vi "catWalkArduinoNew.vi"() -> ()   [LabVIEW 2012]
uses:
  <vilib>/userdefined/High Color/IMAQdx.ctl
  <vilib>/Platform/TimedLoop/XDataNode/timing_clust.ctl
  <vilib>/Platform/TimedLoop/XDataNode/nitl_modes.ctl
  <vilib>/Platform/TimedLoop/XDataNode/wakeup.ctl
  XY Stage/XYStage.llb/GlobalXYStage.vi
  image acquisition/GlobalBaslerCamera.vi
  GlobalStatus.vi
  Cpp Libraries/CatWalkLabviewDLL/labview code/OpenCvGlobals.vi
  GlobalValves.vi
  GlobalLB.vi
  <vilib>/Platform/TimedLoop/XDataNode/XDataNode.xnode
  <vilib>/Platform/TimedLoop/XDataNode/XDNodeRunTimeDep.lvlib
panel:
  out "last time collected fly":u32=479694288
  out "manualStopIndicator":bool=TRUE caption="stop"
  in  "simulated LB status 5":bool[](array[boolean])=[FALSE, FALSE, FALSE, FALSE, FALSE, FALSE]
  in  "simulated LB status 4":bool[](array[boolean])=[FALSE, FALSE, FALSE, FALSE, FALSE, FALSE]
  in  "simulated LB status 3":bool[](array[boolean])=[FALSE, FALSE, FALSE, FALSE, FALSE, FALSE]
  in  "simulated LB status 2":bool[](array[boolean])=[FALSE, FALSE, FALSE, FALSE, FALSE, FALSE]
  in  "autoStop":bool
  in  "stop 2":bool
  in  "Image processing preferences":T1={"scale"=0.5, "elSizeImOpen"=21, "thresholdBinarizationBody"=0.5, "thresholdBinarizationWings"=0.12, "minWingArea"=20000, "quantile"=0.05, "elSizeImOpenIdent1"=15, "elSizeImOpenIdent2"=21, "thresholdBinarizationIdent"=0.65, "elSizeImHMin"=6, "raiseParImHMin"=0.33, "focus limit"=120, "maxAllowedRotation"=30.0, "elSizeImClose"=3, "numIterImClose"=3, "symmetryMinOverlapBody"=95.0, "symmetryMinOverlapWings"=80.0, "thresholdReflectionCheck"=0.99, "elSizeReflection"=7, "maxReflectionArea"=2000, "upSideDownCheck"=260.0}
  out "pre-processing result":T2(plugin-control)
  out "task out":T3(ring)
  out "task":bool=TRUE
  out "status":cluster{"Program status":u32, "message":string}={"Program status"=6618880, "message"="Ready"}
  out "measured flies":i32(slide) caption="Measured flies" scale=0.0..182.0
  out "stop indicator":bool=TRUE
  out "touching rigth border":bool
  in  "image selector":u16(ring) items=["raw image", "single channel", "focus check", "downsampled", "subtraction result", "thresholded", "filtered", "cleaned", "cropped"]
  out "acquiring video":bool
  out "acquired FPS":dbl
  out "processed FPS":dbl
  out "image":T2(plugin-control)
  out "saving background":bool
  in  "Robot Position":T4(radio)
  in  "system info":T5(tab)
  in  "minimum valid\nimages per fly":i32=3 min=1 max=10 step=1
  in  "max time\nin chamber (s)":u32=20
  out "light barriers":bool[](array[boolean])=[FALSE, TRUE]
  in  "loop period (ms)":i64=10
  out "resulting frequency (Hz)":dbl=100.0
  out "valves status":bool[](array[boolean])
  in  "resave BG time":u32=120
  in  "milliseconds to wait\nafter detection":u32
  in  "max number of\nimages per fly":i32=100
  in  "activate flies time interval (s)":u32=30
  out "done sorting":bool
  in  "sort one by one":bool
  in  "max time \nin chamber after\ndetection (s)":u32=25
  in  "inactivity alarm time interval (s)":u32=180
  in  "valve open time blow back":u32=1500
  in  "valve open time eject":u32=2000
  in  "valve open time keep":u32=5000
  in  "open valve":bool
  in  "valve close":bool[](array[boolean])=[FALSE, FALSE, FALSE, FALSE, FALSE, FALSE, FALSE, FALSE]
  in  "valve to hangar":bool[](array[boolean])=[TRUE, FALSE, TRUE, FALSE, FALSE, FALSE, FALSE, FALSE]
  in  "valve back":bool[](array[boolean])=[TRUE, FALSE, FALSE, FALSE, FALSE, FALSE, FALSE, FALSE]
  in  "valve eject":bool[](array[boolean])=[FALSE, TRUE, TRUE, FALSE, FALSE, FALSE, FALSE, FALSE]
  in  "valves puffed":bool[](array[boolean])=[FALSE, FALSE, TRUE, FALSE, FALSE, FALSE, FALSE, FALSE]
  in  "numPuffs keep":i32=3 min=1 max=10
  in  "numPuffs eject":i32=5
  in  "numPuffs blowback":i32=2 min=1 max=10
  in  "waitms before puff":u32=300
  in  "valve open time activate":u32=1000
  in  "number of\npuffs for scaring":i32=2
  in  "valve open time pre":u32=400
  in  "numPuffs eject pre":i32=3
  in  "valve open time blow back 2":u32=1000
  in  "valve open time activate pre":u32=1000
  in  "USB COM port":refnum<visa-resource-name>="COM3"
  in  "robot limits":T6={"xmin"=-16850, "xmax"=-1660, "ymin"=-15485, "ymax"=-550}
  in  "Motor high speed":i32=5000
  in  "Motor low speed":i32=100
  in  "Motor acc":i32=500
  in  "gate 0 closed blowing":u16=1380
  in  "fly trap open":u16=1490
  in  "fly trap close":u16=1490
  in  "fly ejector open":u16=1350
  in  "fly ejector close":u16=900
  in  "fly sieve hangar":u16=1390
  in  "gate 0 closed":u16=1390
  in  "gate 0 open":u16=1470
  in  "fly sieve back":u16=1680
  in  "fly sieve odour":u16=1140
  in  "bottle positions":u16[](array[numeric])=[1115, 1210, 1290]
  in  "shakeSpan":i8 max=63 step=1
  in  "gate 0 open blowing":u16=1470
  in  "free gate after keeping":bool=TRUE
  in  "disable servo delay (ms)":u32=200
  in  "fly ejector semi close":u16=1150
  in  "numShakes":i32=3
  in  "shake speed":u32=50
  in  "insensitivity time (ms)":u32=2000
  in  "camera controls":T8={"Camera Name"="cam0", "exposure time (us)"=600, "GainRaw"=200, "Red balance"=75, "Green balance"=80, "Blue balance"=64}
  in  "image format controls":T9={"Pixel Format"="YUV 422 Packed", "width"=2448, "height"=900, "sub image height"=600, "sub image width"=1500}
  in  "im proc controls":T10={"Color Plane"=2, "downsampling"=64, "Filter"=enum."AutoM", "Number of Erosions"=1, "Focus threshold"=20.0, "Focus std threshold"=0.0, "background\nsubtraction"=TRUE, "Threshold"=40} {"Threshold" scale=0.0..255.0; "downsampling" min=1 max=128; "Color Plane" items=["Red", "Green", "Blue", "Hue", "Saturation", "Luminance", "Value", "Intensity"]}
  in  "adjust image":bool
  out "filled buffer":i32(slide) max=20 scale=0.0..500.0
  in  "buffer size":i32=500
  in  "simulate LB":bool
  in  "simulated LB status":bool[](array[boolean])=[FALSE, FALSE, FALSE, FALSE, FALSE, FALSE]
  out "events check loop":i32=163273
  in  "debugOpenCV":bool
  in  "keep all flies":bool
  out "numCycles":i32=198986
  in  "experiment name":string="L1S4fb"
  in  "data path":path=path "Y:/WingXDataRemote"
  in  "temp path":path=path "C:/wingXTemp"
  in  "sounds":T11={"welcome sound"=path "C:/Users/wingX/Documents/WingXSVN/labview/daq test/sounds/welcome.wav", "play welcome"=FALSE, "got fly sound"=path "C:/Users/wingX/Documents/WingXSVN/labview/daq test/sounds/gotFly.wav", "play got fly"=FALSE, "discard sound"=path "C:/Users/wingX/Documents/WingXSVN/labview/daq test/sounds/blowingback.wav", "play discard"=FALSE, "finish sound"=path "C:/Users/wingX/Documents/WingXSVN/labview/daq test/sounds/done.wav", "play finish"=TRUE, "inactivity alarm sound"=path "C:/Users/wingX/Documents/WingXSVN/labview/daq test/sounds/inactivity.wav", "play inactivity\nalarm"=TRUE}
  in  "stop":bool
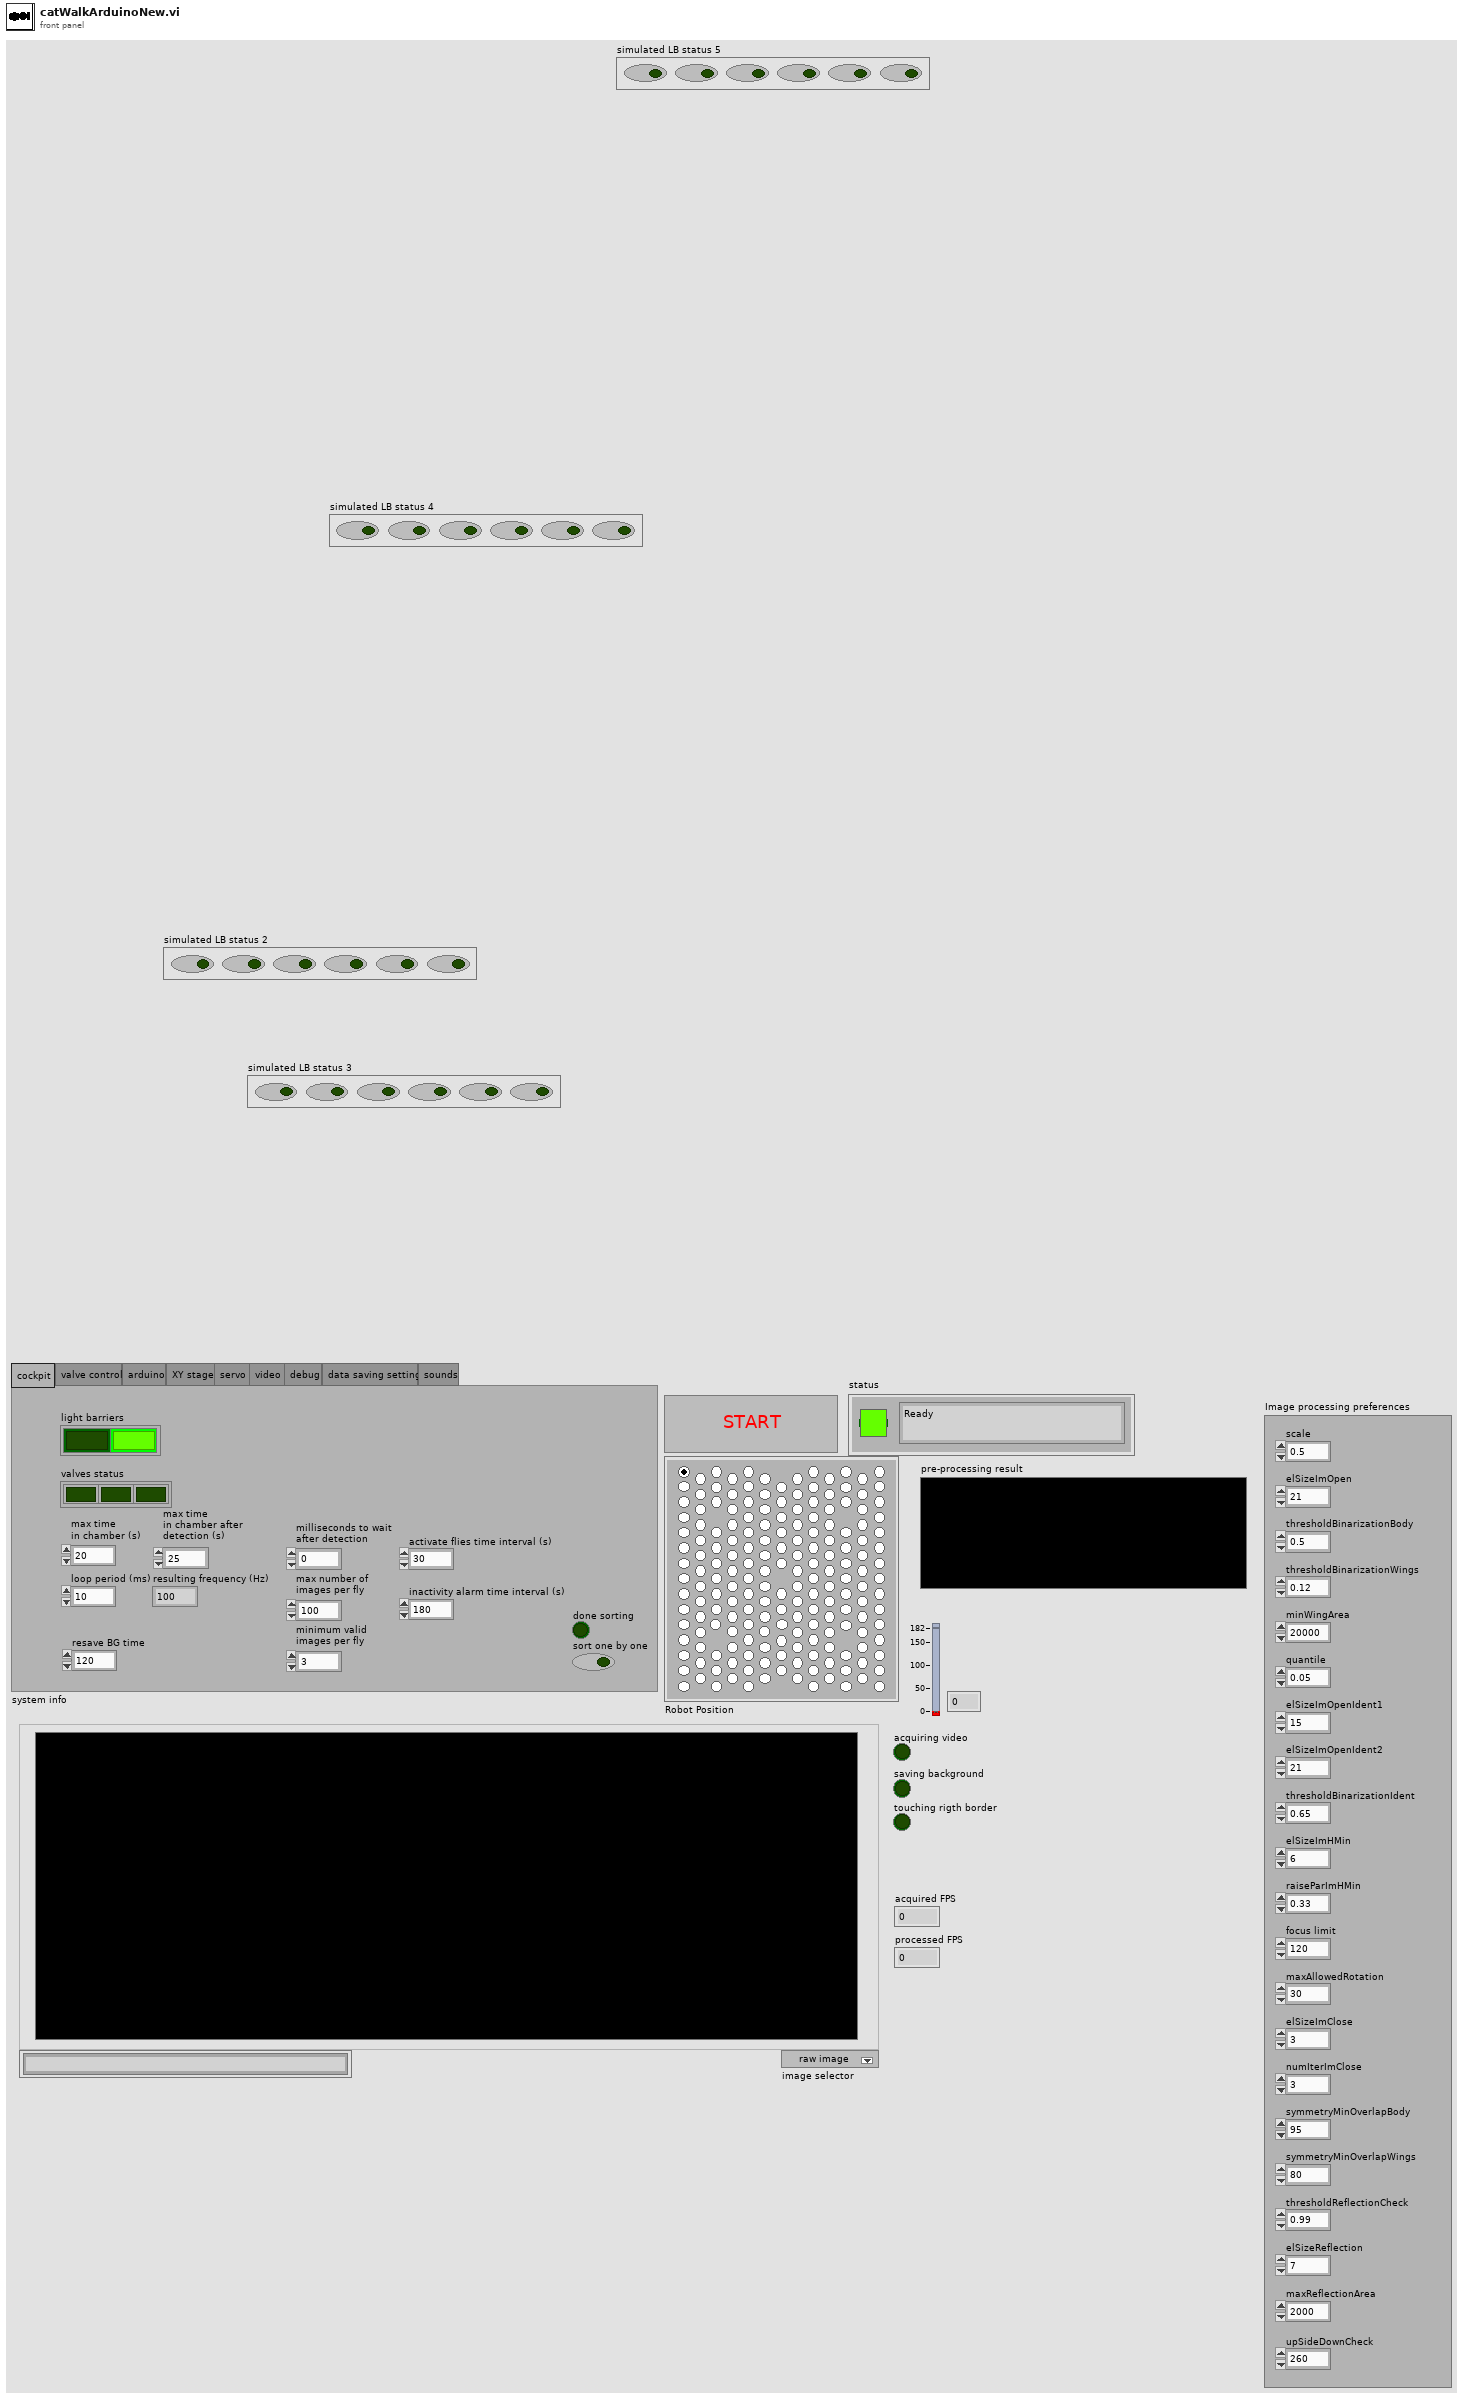
[diagram p1: front panel]
types:
  T1 = cluster{"scale":sgl, "elSizeImOpen":i32, "thresholdBinarizationBody":sgl, "thresholdBinarizationWings":sgl, "minWingArea":i32, "quantile":sgl, "elSizeImOpenIdent1":i32, "elSizeImOpenIdent2":i32, "thresholdBinarizationIdent":sgl, "elSizeImHMin":i32, "raiseParImHMin":sgl, "focus limit":i32, "maxAllowedRotation":sgl, "elSizeImClose":i32, "numIterImClose":i32, "symmetryMinOverlapBody":sgl, "symmetryMinOverlapWings":sgl, "thresholdReflectionCheck":sgl, "elSizeReflection":i32, "maxReflectionArea":i32, "upSideDownCheck":sgl}
  T2 = typedef "IMAQ Image.ctl" = refnum<image>
  T3 = enum16{"waiting for fly", "closing gate", "fly in chamber", "taking decision", "keeping the fly", "blowing back", "activate flies"}
  T4 = enum32{"Radio Selection 1", "Radio Selection 2", "Radio Selection 3", "Radio Selection 5", "Radio Selection 6", "Radio Selection 8", "Radio Selection 13", "Radio Selection 14", "Radio Selection 15", "Radio Selection 16", "Radio Selection 17", "Radio Selection 18", "Radio Selection 7", "Radio Selection 9", "Radio Selection 10", "Radio Selection 11", "Radio Selection 12", "Radio Selection 19", "Radio Selection 20", "Radio Selection 21", "Radio Selection 22", "Radio Selection 23", "Radio Selection 24", "Radio Selection 25", "Radio Selection 26", "Radio Selection 27", "Radio Selection 28", "Radio Selection 29", "Radio Selection 30", "Radio Selection 31", "Radio Selection 32", "Radio Selection 33", "Radio Selection 34", "Radio Selection 35", "Radio Selection 36", "Radio Selection 37", "Radio Selection 38", "Radio Selection 39", "Radio Selection 40", "Radio Selection 42", "Radio Selection 43", "Radio Selection 44", "Radio Selection 46", "Radio Selection 41", "Radio Selection 45", "Radio Selection 47", "Radio Selection 48", "Radio Selection 49", "Radio Selection 50", "Radio Selection 51", "Radio Selection 52", "Radio Selection 53", "Radio Selection 54", "Radio Selection 55", "Radio Selection 56", "Radio Selection 57", "Radio Selection 58", "Radio Selection 59", "Radio Selection 60", "Radio Selection 61", "Radio Selection 62", "Radio Selection 63", "Radio Selection 64", "Radio Selection 65", "Radio Selection 66", "Radio Selection 67", "Radio Selection 68", "Radio Selection 69", "Radio Selection 70", "Radio Selection 71", "Radio Selection 72", "Radio Selection 73", "Radio Selection 74", "Radio Selection 75", "Radio Selection 76", "Radio Selection 77", "Radio Selection 78", "Radio Selection 79", "Radio Selection 80", "Radio Selection 81", "Radio Selection 82", "Radio Selection 83", "Radio Selection 84", "Radio Selection 85", "Radio Selection 86", "Radio Selection 87", "Radio Selection 88", "Radio Selection 89", "Radio Selection 4", "Radio Selection 90", "Radio Selection 91", "Radio Selection 92", "Radio Selection 93", "Radio Selection 94", "Radio Selection 95", "Radio Selection 96", "Radio Selection 97", "Radio Selection 98", "Radio Selection 99", "Radio Selection 100", "Radio Selection 101", "Radio Selection 102", "Radio Selection 103", "Radio Selection 104", "Radio Selection 105", "Radio Selection 106", "Radio Selection 107", "Radio Selection 108", "Radio Selection 109", "Radio Selection 110", "Radio Selection 111", "Radio Selection 112", "Radio Selection 113", "Radio Selection 114", "Radio Selection 115", "Radio Selection 116", "Radio Selection 117", "Radio Selection 118", "Radio Selection 119", "Radio Selection 120", "Radio Selection 121", "Radio Selection 122", "Radio Selection 123", "Radio Selection 124", "Radio Selection 125", "Radio Selection 126", "Radio Selection 127", "Radio Selection 128", "Radio Selection 129", "Radio Selection 130", "Radio Selection 131", "Radio Selection 132", "Radio Selection 133", "Radio Selection 134", "Radio Selection 135", "Radio Selection 136", "Radio Selection 137", "Radio Selection 138", "Radio Selection 139", "Radio Selection 140", "Radio Selection 141", "Radio Selection 142", "Radio Selection 143", "Radio Selection 144", "Radio Selection 145", "Radio Selection 146", "Radio Selection 147", "Radio Selection 148", "Radio Selection 149", "Radio Selection 150", "Radio Selection 151", "Radio Selection 152", "Radio Selection 153", "Radio Selection 154", "Radio Selection 155", "Radio Selection 156", "Radio Selection 157", "Radio Selection 158", "Radio Selection 159", "Radio Selection 160", "Radio Selection 161", "Radio Selection 162", "Radio Selection 163", "Radio Selection 164", "Radio Selection 165", "Radio Selection 166", "Radio Selection 167", "Radio Selection 168", "Radio Selection 169", "Radio Selection 170", "Radio Selection 171", "Radio Selection 172", "Radio Selection 173", "Radio Selection 174", "Radio Selection 175", "Radio Selection 176", "Radio Selection 177", "Radio Selection 178", "Radio Selection 179", "Radio Selection 180", "Radio Selection 181", "Radio Selection 182"}
  T5 = enum32{"cockpit", "valve control", "arduino", "XY stage", "servo", "video", "debug", "data saving settings", "sounds"}
  T6 = cluster{"xmin":i32, "xmax":i32, "ymin":i32, "ymax":i32}
  T7 = typedef "IMAQdx.ctl" = refnum<k21>
  T8 = cluster{"Camera Name":T7, "exposure time (us)":u32, "GainRaw":i64, "Red balance":i64, "Green balance":i64, "Blue balance":i64}
  T9 = cluster{"Pixel Format":string, "width":u32, "height":u32, "sub image height":u32, "sub image width":u32}
  T10 = cluster{"Color Plane":i32, "downsampling":i32, "Filter":enum32{"AutoM", "Close", "Dilate", "Erode", "Gradient", "Gradient out", "Gradient in", "Hit miss", "Open", "PClose", "POpen", "Thick", "Thin"}, "Number of Erosions":i32, "Focus threshold":sgl, "Focus std threshold":sgl, "background\nsubtraction":bool, "Threshold":u8}
  T11 = cluster{"welcome sound":path, "play welcome":bool, "got fly sound":path, "play got fly":bool, "discard sound":path, "play discard":bool, "finish sound":path, "play finish":bool, "inactivity alarm sound":path, "play inactivity\nalarm":bool}
  T12 = typedef "XDNodeRunTimeDep.lvlib/timing_clust.ctl" = cluster{"Expected End [f-1]":u64, "Actual End [f-1]":u64, "Finished Late? [f-1]":bool, "Expected End [i-1]":u64, "Actual End [i-1]":u64, "Finished Late? [i-1]":bool, "Expected Start [i]":u64, "Actual Start [i]":u64, "Expected Start [f]":u64, "Actual Start [f]":u64, "Source Name":string, "Structure Name":string, "Period":i64, "Deadline":i64, "Offset":i64, "Start":i64, "Priority":i32, "Timeout":i32, "Mode":T13, "Wakeup Reason":T14, "Error":errorcluster, "Source Type":string, "Secondary Source Type":string, "Global End Time":u64, "Global Start Time":u64, "Frame Duration":u64, "Iteration Duration":u64, "Assigned CPU":i32, "I/O Scan Engine Mode":u32}
  T13 = typedef "XDNodeRunTimeDep.lvlib/nitl_modes.ctl" = enum32{"No Change", "Process missed periods, maintain original phase", "Discard missed periods, maintain original phase", "Process missed periods, ignore original phase", "Discard missed periods, ignore original phase"}
  T14 = typedef "XDNodeRunTimeDep.lvlib/wakeup.ctl" = enum32{"Normal", "Aborted", "Asynchronous wakeup", "Timing source error", "Timed loop error", "Timeout"}
  T15 = enum16{"Left Button", "Center Button", "Right Button", "Window Close"}
  T16 = typedef "Semaphore RefNum" = refnum<k1>
  T17 = enum8{"Enabled", "Disabled", "Disabled and Grayed Out"}
  T18 = cluster{"raw":T2, "single channel":T2, "focus check":T2, "downsampled":T2, "subtraction":T2, "thresholded":T2, "filtered":T2, "cleaned":T2, "cropped":T2}
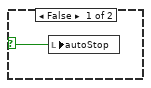
[diagram p2: hidden frame]
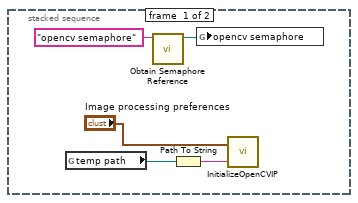
[diagram p4: hidden frame]
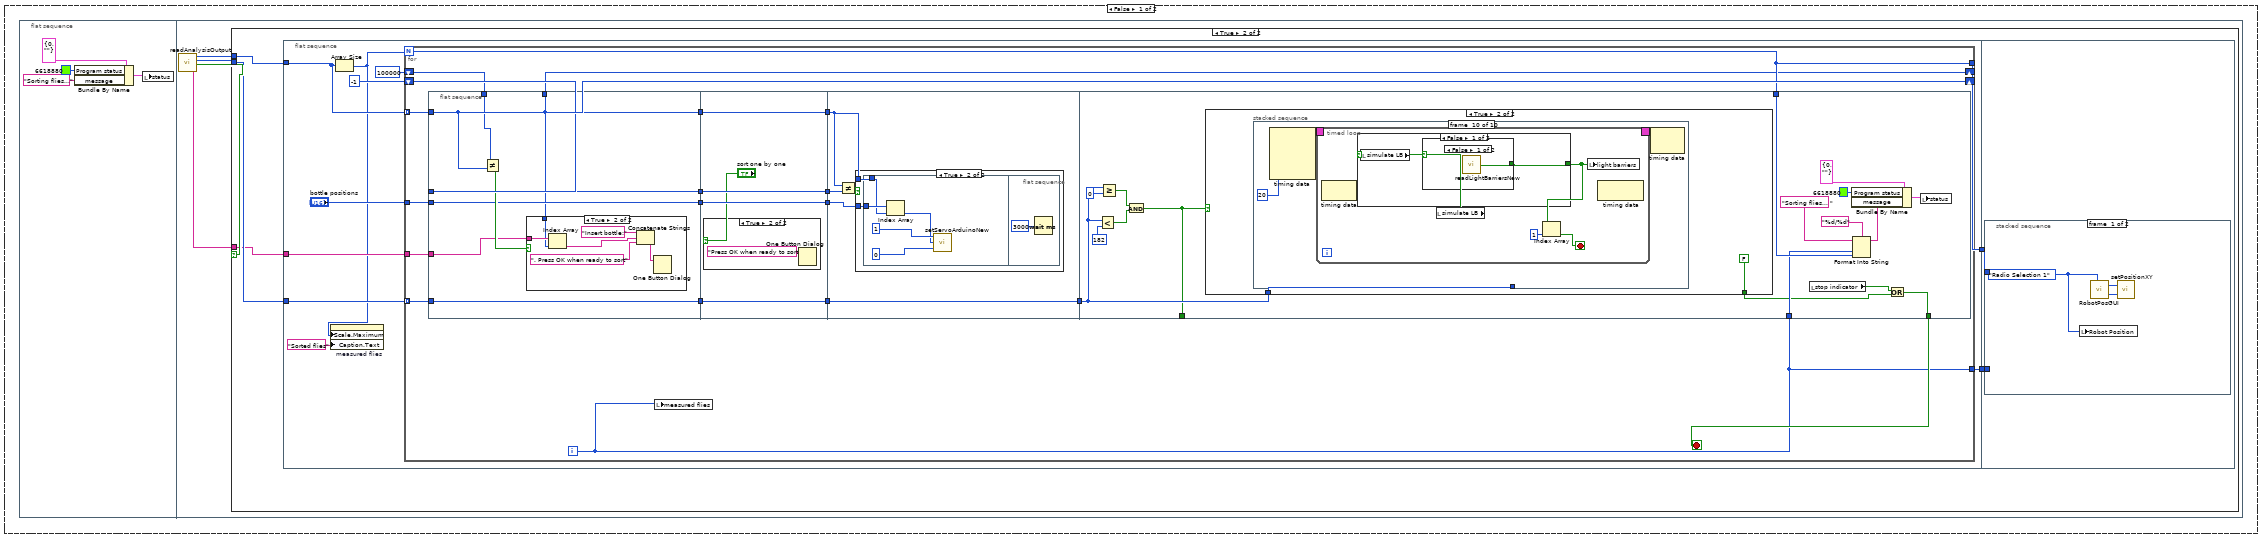
[diagram p6: hidden frame]
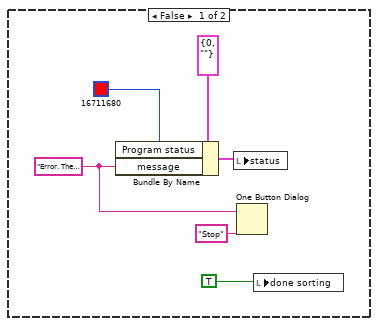
[diagram p7: hidden frame]
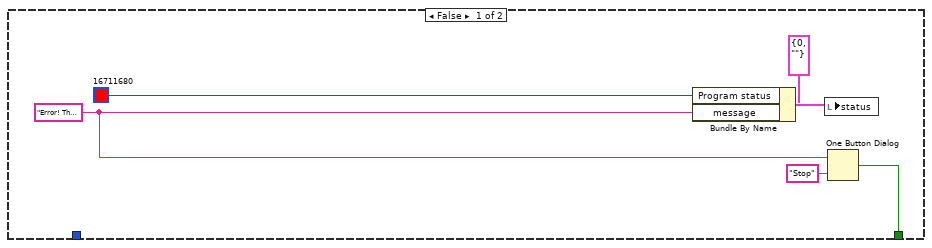
[diagram p11: hidden frame]
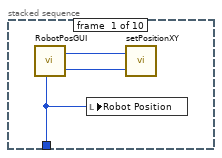
[diagram p12: hidden frame]
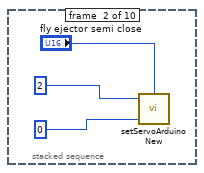
[diagram p13: hidden frame]
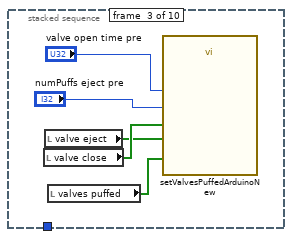
[diagram p14: hidden frame]
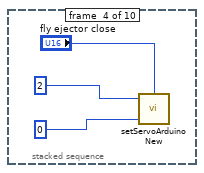
[diagram p15: hidden frame]
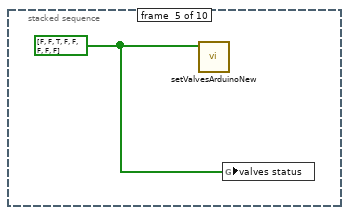
[diagram p16: hidden frame]
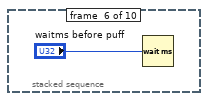
[diagram p17: hidden frame]
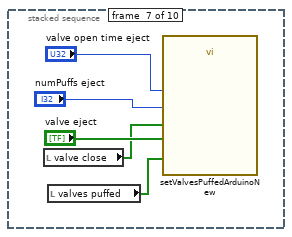
[diagram p18: hidden frame]
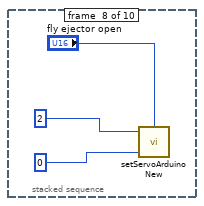
[diagram p19: hidden frame]
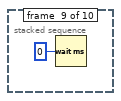
[diagram p20: hidden frame]
diagram:
  n1 = while {
    stop <- "stop 2" stop-if-true
    n2 = flat-sequence {
      tunnel: ["loop period (ms)"] -> w3
      tunnel: w3 -> [w80]
      tunnel: [w80] -> w2
      tunnel: w2 -> [w85]
      frame #0 {
        n3 = node-c288(i64 10 ("Period")) -> (w10:T12)  [unwired: 3 in]
        n4 = timed-loop {
          timing: w10 -> [_]
          timing-out: [_] -> w9
          stop <- w13 stop-if-true
          n5 = node-c288() -> ()  [unwired: 1 in, 1 out]
          n6 = local read "Robot Position"() -> (w12:T4)
          n7 = global write "GlobalXYStage.vi" "Robot Position"(w12) -> ()
          n8 = local write "measured flies"(w12) -> ()
          n9 = local read "stop"() -> (w13:bool)
          n10 = node-c288() -> ()  [unwired: 1 in, 1 out]
        }
        n11 = property on="stop" class="Bool (strict)"("BoolText.Text"="START" ("Boolean Text.Text")) -> ()  [unwired: 2 in, 2 out]
        n12 = Bundle By Name(cluster=cluster{"Program status":u32, "message":string} {"Program status"=0, "message"=""} ("status 2"), "Program status"=u32 6618880, "message"="Ready") -> (w5:cluster{"Program status":u32, "message":string})
        n13 = local write "status"(w5) -> ()
        n14 = node-c288(w9) -> ()  [unwired: 1 out]
      }
      frame #1 {
        w20 = FALSE ("stop indicator")
        # "init arduino and close gate"
        n15 = flat-sequence {
          frame #0 {
            n16 = call "initArduinoNew.vi"("VISA resource"="USB COM port") -> ()
          }
          frame #1 {
            n17 = local read "fly ejector open"() -> (w30:u16)
            n18 = local read "gate 0 closed"() -> (w35:u16)
            n19 = call "setServoArduinoNew.vi"("speed"=u8 0, "Pulse Width in uS"=w35, "servo id"=u8 0 ("channel")) -> ()
            n20 = call "setServoArduinoNew.vi"("speed"=u8 0, "Pulse Width in uS"=w30, "servo id"=u8 2 ("channel")) -> ()
          }
          frame #2 {
            n21 = Wait (ms)(milliseconds to wait=u32 500) -> ()  [unwired: 1 out]
          }
          frame #3 {
            n22 = call "disableServosArduinoNew.vi"() -> ()  [unwired: 1 in]
          }
        }
        n23 = property on="stop" class="Bool (strict)"("Value"=FALSE ("stop")) -> ()  [unwired: 2 in, 2 out]
        n24 = property on="stop" class="Bool (strict)"("BoolText.Text"="STOP" ("Boolean Text.Text")) -> ()  [unwired: 2 in, 2 out]
        n25 = local write "stop indicator"(w20) -> ()
        n26 = Bundle By Name(cluster=cluster{"Program status":u32, "message":string} {"Program status"=0, "message"=""} ("status 2"), "Program status"=u32 16776960, "message"="Initializing...") -> (→"status":cluster{"Program status":u32, "message":string})
        n27 = property on="measured flies" class="Slide (strict)"("Scale.Maximum"=182 ("Scale.Range:Maximum"), "Caption.Text"="") -> ()  [unwired: 2 in, 2 out]
        "done sorting" <- w20
      }
      frame #2 {
        n28 = local read "adjust image"() -> (w54:bool)
        n29 = global write "GlobalBaslerCamera.vi" "temp path"("temp path") -> ()
        n30 = global write "GlobalBaslerCamera.vi" "data path"("data path") -> ()
        n31 = Divide(x=i64 1000, y="loop period (ms)") -> (x/y=→"resulting frequency (Hz)":dbl)
        n32 = call <vilib>:"Three Button Dialog.vi"("Right Button Text (\"Cancel\")"="Sort Flies" ("F button name (\"Cancel\")"), "Center Button Text (\"No\")"="Measure flies starting from current position" ("T button name (\"OK\")"), "Left Button Text (\"Yes\")"="Measure flies" ("T button name (\"OK\")"), "message"="WELCOME TO THE FLY CATWALK\n\nWhat do you want to do?") -> ("Which Button?"=w38:T15)  [unwired: 7 in]
        n33 = Equal?(x=T15."Center Button", y=w38) -> (x = y?=w42:bool)
        n34 = global write "GlobalBaslerCamera.vi" "adjust image"(w54) -> ()
        n35 = call "initXYStage.vi"("Motor high speed"="Motor high speed", "restart from\ncurrent position"=w42, "Motor acc"="Motor acc", "Motor low speed"="Motor low speed", "robot limits"="robot limits") -> ("Robot Position"=w40:T4)
        "measured flies" <- w40
        n36 = global write "GlobalStatus.vi" "hangar full"(FALSE ("hangar full")) -> ()
        n37 = Less?(x=w38, y=T15."Right Button") -> (x < y?=w44:bool)
        "task" <- w44
        n38 = case shown="True" w44 {
          frame False {
          }
          frame True {
            n39 = stacked-sequence {
              frame #0 {
                n40 = global read "GlobalBaslerCamera.vi" "temp path"() -> (w67:path)
                n41 = call <vilib>:"Obtain Semaphore Reference.vi"("name (unnamed)"="opencv semaphore") -> ("semaphore"=w64:T16)  [unwired: 4 in, 2 out]
                n42 = Path To String(path=w67) -> (string=w66:string)
                n43 = global write "OpenCvGlobals.vi" "opencv semaphore"(w64) -> ()
                n44 = call "InitializeOpenCVIP.vi"("dataDirectory"=w66, "Image processing preferences"="Image processing preferences") -> ()  [unwired: 1 out]
              }
              frame #1 {
                n45 = local read "im proc controls"() -> (w69:T10)
                n46 = call "initBaslerCamera.vi"("buffer size"="buffer size", "camera controls"="camera controls", "im proc controls"=w69, "image format controls"="image format controls") -> ()  [unwired: 4 in]
                n47 = property on="filled buffer" class="Slide (strict)"("Scale.Maximum"="buffer size") -> ()  [unwired: 2 in, 2 out]
              }
            }
          }
        }
        n48 = Equal?(x=T15."Window Close", y=w38) -> (x = y?=w39:bool)
        n49 = global write "GlobalBaslerCamera.vi" "experiment name"("experiment name") -> ()
        n50 = case shown="True" w39 {
          selector: w39 -> [w61 w62]
          frame False {
            n51 = local write "autoStop"(w61) -> ()
          }
          frame True {
            n52 = local write "autoStop"(w62) -> ()
          }
        }
        n53 = local write "Robot Position"(w40) -> ()
      }
      frame #3 {
        w79 = T17."Disabled and Grayed Out" ("Disabled")
        n54 = global write "OpenCvGlobals.vi" "isDebug"("debugOpenCV") -> ()
        n55 = local read "fly sieve odour"() -> (w76:u16)
        n56 = local read "gate 0 closed"() -> (w72:u16)
        n57 = property on="loop period (ms)" class="DigNum (strict)"("DisabledEnum"=w79) -> ()  [unwired: 2 in, 2 out]
        n58 = property on="image format controls" class="Clust (strict)"("DisabledEnum"=w79) -> ()  [unwired: 2 in, 2 out]
        n59 = property on="camera controls" class="Clust (strict)"("DisabledEnum"=w79) -> ()  [unwired: 2 in, 2 out]
        n60 = property on="temp path" class="Path"("DisabledEnum"=w79) -> ()  [unwired: 2 in, 2 out]
        n61 = property on="data path" class="Path"("DisabledEnum"=w79) -> ()  [unwired: 2 in, 2 out]
        n62 = call "setServoArduinoNew.vi"("speed"=u8 0, "Pulse Width in uS"=w76, "servo id"=u8 1 ("channel")) -> ()
        n63 = call "setServoArduinoNew.vi"("speed"=u8 0, "Pulse Width in uS"=w72, "servo id"=u8 0 ("channel")) -> ()
      }
      frame #4 {
        n64 = node-c288(i64 100 ("Period")) -> (w84:T12)  [unwired: 3 in]
        n65 = local read "task"() -> (w81:bool)
        n66 = timed-loop {
          timing: w84 -> [_]
          timing-out: [_] -> w83
          stop <- w92 stop-if-true
          n67 = node-c288() -> ()  [unwired: 1 in, 1 out]
          n68 = local read "done sorting"() -> (w89:bool)
          n69 = global read "GlobalStatus.vi" "hangar full"() -> (w90:bool)
          n70 = Compound Arithmetic op=OR("autoStop", w90, w89, "stop") -> (w92:bool)
          "stop indicator" <- w92
          n71 = call "disableServosArduinoNew.vi"("delay (ms)"="disable servo delay (ms)") -> ()
          n72 = node-c288() -> ()  [unwired: 1 in, 1 out]
          "manualStopIndicator" <- "stop"
        }
        n73 = case shown="True" w81 {
          frame False {
          }
          frame True {
            n74 = property on="measured flies" class="Slide (strict)"("Caption.Text"="Measured flies" ("Label.Text")) -> ()  [unwired: 2 in, 2 out]
          }
        }
        n75 = node-c288(w83) -> ()  [unwired: 1 out]
        n76 = case shown="True" w81 {
          tunnel: w85 -> [_ w269]
          frame False {
            n77 = flat-sequence {
              frame #0 {
                n78 = Bundle By Name(cluster=cluster{"Program status":u32, "message":string} {"Program status"=0, "message"=""} ("status 2"), "Program status"=u32 6618880, "message"="Sorting flies...") -> (w100:cluster{"Program status":u32, "message":string})
                n79 = local write "status"(w100) -> ()
              }
              frame #1 {
                n80 = call "readAnalysisOutput.vi"() -> ("bottle number"=w106:i64[], "fly number"=w105:i64[], "folder exists"=w104:bool, "bottle label"=w103:string[])  [unwired: 1 in]
                n81 = case shown="True" w104 {
                  tunnel: w106 -> [_ w117]
                  tunnel: w105 -> [_ w116]
                  tunnel: w103 -> [_ w113]
                  frame False {
                    w109 = "Error. The selected directory does not contain an Analysisoutpu.txt file. It may not be analized yet. The program will stop immediately" ("message")
                    n82 = Bundle By Name(cluster=cluster{"Program status":u32, "message":string} {"Program status"=0, "message"=""} ("status 2"), "Program status"=u32 16711680, "message"=w109) -> (w111:cluster{"Program status":u32, "message":string})
                    n83 = local write "status"(w111) -> ()
                    n84 = One Button Dialog(message=w109, button name ("OK")="Stop") -> ()  [unwired: 1 out]
                    n85 = local write "done sorting"(TRUE) -> ()
                  }
                  frame True {
                    n86 = flat-sequence {
                      tunnel: w117 -> [w127]
                      tunnel: w116 -> [w124]
                      tunnel: [w123] -> w115
                      tunnel: [w122] -> w114
                      tunnel: w113 -> [w121]
                      tunnel: w115 -> [w248]
                      tunnel: w114 -> [w247]
                      frame #0 {
                        n87 = Array Size(array=w127) -> (size(s)=w119:i32)
                        n88 = property on="measured flies" class="Slide (strict)"("Scale.Maximum"=w119, "Caption.Text"="Sorted flies" ("Label.Text")) -> ()  [unwired: 2 in, 2 out]
                        n89 = for {
                          N: w119 -> [w141]
                          tunnel: w127 -> [w146] mode=indexing
                          shift-right: [w146] -> _
                          shift-left: i64 -1 -> [w145]
                          tunnel: "bottle positions" -> [w144]
                          tunnel: w124 -> [w142] mode=indexing
                          tunnel: [w128] -> w123
                          tunnel: [w141] -> w122
                          shift-right: [w129] -> _
                          shift-left: i64 100000 -> [w131]
                          tunnel: w121 -> [w130]
                          i -> [w128]
                          stop <- w136 stop-if-true
                          n90 = flat-sequence {
                            tunnel: w142 -> [w148]
                            tunnel: w144 -> [w149]
                            tunnel: w145 -> [w153]
                            tunnel: w146 -> [w147]
                            tunnel: [w147] -> w135
                            tunnel: [w153] -> w134
                            tunnel: [w149] -> w133
                            tunnel: [w148] -> w132
                            tunnel: w131 -> [w152]
                            tunnel: w130 -> [w150]
                            tunnel: [w147] -> w129
                            tunnel: [w164] -> w140
                            tunnel: [w163] -> w139
                            tunnel: [w162] -> w138
                            tunnel: [w161] -> w137
                            tunnel: w135 -> [w164]
                            tunnel: w134 -> [w163]
                            tunnel: w133 -> [w162]
                            tunnel: w132 -> [w161]
                            tunnel: [w166] -> w143
                            tunnel: w140 -> [w167]
                            tunnel: w139 -> [w169]
                            tunnel: w138 -> [w168]
                            tunnel: w137 -> [w166]
                            tunnel: [w190] -> _
                            tunnel: w143 -> [w194]
                            tunnel: w128 -> [w182]
                            tunnel: w141 -> [w185]
                            tunnel: [w179] -> w136
                            frame #0 {
                              n91 = Not Equal?(x=w152, y=w147) -> (x != y?=w151:bool)
                              n92 = case shown="True" w151 {
                                tunnel: w150 -> [_ w157]
                                tunnel: w147 -> [_ w156]
                                frame False {
                                }
                                frame True {
                                n93 = Index Array(array=w157, index=w156) -> (element=w155:string)
                                n94 = Concatenate Strings("Insert bottle:" ("message"), w155, ". Press OK when ready to sort" ("message")) -> (w154:string)
                                n95 = One Button Dialog(message=w154) -> ()  [unwired: 1 in, 1 out]
                                }
                              }
                            }
                            frame #1 {
                              n96 = case shown="True" "sort one by one" {
                                frame False {
                                }
                                frame True {
                                n97 = One Button Dialog(message="Press OK when ready to sort") -> ()  [unwired: 1 in, 1 out]
                                }
                              }
                            }
                            frame #2 {
                              n98 = Not Equal?(x=w167, y=w169) -> (x != y?=w170:bool)
                              n99 = case shown="True" w170 {
                                tunnel: w168 -> [_ w172]
                                tunnel: w167 -> [_ w171]
                                frame False {
                                }
                                frame True {
                                n100 = flat-sequence {
                                tunnel: w172 -> [w175]
                                tunnel: w171 -> [w174]
                                frame #0 {
                                n101 = Index Array(array=w175, index=w174) -> (element=w173:u16)
                                n102 = call "setServoArduinoNew.vi"("speed"=u8 0, "Pulse Width in uS"=w173, "servo id"=u8 1 ("channel")) -> ()
                                }
                                frame #1 {
                                n103 = Wait (ms)(milliseconds to wait=u32 3000) -> ()  [unwired: 1 out]
                                }
                                }
                                }
                              }
                            }
                            frame #3 {
                              n104 = Less?(x=w194, y=i64 182) -> (x < y?=w192:bool)
                              n105 = Greater Or Equal?(x=w194, y=i64 0) -> (x >= y?=w191:bool)
                              n106 = And(x=w191, y=w192) -> (x .and. y?=w190:bool)
                              n107 = case shown="True" w190 {
                                tunnel: w194 -> [_ w203]
                                tunnel: [w196 FALSE ("true")] -> w181
                                frame False {
                                w198 = "Error! The analysis output file contains invalid data.  The program will terminate immediately." ("message")
                                n108 = Bundle By Name(cluster=cluster{"Program status":u32, "message":string} {"Program status"=0, "message"=""} ("status 2"), "Program status"=u32 16711680, "message"=w198) -> (w200:cluster{"Program status":u32, "message":string})
                                n109 = local write "status"(w200) -> ()
                                n110 = One Button Dialog(message=w198, button name ("OK")="Stop") -> (true=w196:bool)
                                }
                                frame True {
                                n111 = stacked-sequence {
                                tunnel: w203 -> [w204 _ _ _ _ _ _ _ _ _]
                                frame #0 {
                                n112 = call "RobotPosGUI.vi"("Robot Position"=w204) -> ("X position"=w206:i32, "Y position"=w205:i32)  [unwired: 4 in]
                                n113 = local write "Robot Position"(w204) -> ()
                                n114 = call "setPositionXY.vi"("Y Position"=w205, "X Position"=w206) -> ()  [unwired: 1 in]
                                }
                                frame #1 {
                                n115 = call "setServoArduinoNew.vi"("speed"=u8 0, "Pulse Width in uS"="fly ejector semi close", "servo id"=u8 2 ("channel")) -> ()
                                }
                                frame #2 {
                                n116 = local read "valve close"() -> (w213:bool[])
                                n117 = local read "valve eject"() -> (w210:bool[])
                                n118 = local read "valves puffed"() -> (w212:bool[])
                                n119 = call "setValvesPuffedArduinoNew.vi"("valve data puffed"=w212, "valve data close"=w213, "valve data open"=w210, "milliseconds to wait"="valve open time pre", "numPuffs"="numPuffs eject pre") -> ()  [unwired: 7 in]
                                }
                                frame #3 {
                                n120 = call "setServoArduinoNew.vi"("speed"=u8 0, "Pulse Width in uS"="fly ejector close", "servo id"=u8 2 ("channel")) -> ()
                                }
                                frame #4 {
                                w218 = bool[] [FALSE, FALSE, TRUE, FALSE, FALSE, FALSE, FALSE, FALSE] ("valve data open")
                                n121 = call "setValvesArduinoNew.vi"("valve data"=w218) -> ()  [unwired: 11 in]
                                n122 = global write "GlobalValves.vi" "valves status"(w218) -> ()
                                }
                                frame #5 {
                                n123 = Wait (ms)(milliseconds to wait="waitms before puff") -> ()  [unwired: 1 out]
                                }
                                frame #6 {
                                n124 = local read "valve close"() -> (w222:bool[])
                                n125 = local read "valves puffed"() -> (w221:bool[])
                                n126 = call "setValvesPuffedArduinoNew.vi"("valve data puffed"=w221, "valve data close"=w222, "valve data open"="valve eject", "milliseconds to wait"="valve open time eject", "numPuffs"="numPuffs eject") -> ()  [unwired: 7 in]
                                }
                                frame #7 {
                                n127 = call "setServoArduinoNew.vi"("speed"=u8 0, "Pulse Width in uS"="fly ejector open", "servo id"=u8 2 ("channel")) -> ()
                                }
                                frame #8 {
                                n128 = Wait (ms)(milliseconds to wait=u32 0) -> ()  [unwired: 1 out]
                                }
                                frame #9 {
                                n129 = node-c288(i64 20 ("Period")) -> (w231:T12)  [unwired: 3 in]
                                n130 = timed-loop {
                                timing: w231 -> [_]
                                timing-out: [_] -> w230
                                stop <- w234 stop-if-true
                                n131 = node-c288() -> ()  [unwired: 1 in, 1 out]
                                n132 = local read "simulate LB"() -> (w233:bool)
                                n133 = case shown="False" w233 {
                                tunnel: [w236 "simulated LB status 2"] -> w232
                                frame False {
                                n134 = local read "simulate LB"() -> (w237:bool)
                                n135 = case shown="False" w237 {
                                tunnel: [w238 "simulated LB status 5"] -> w236
                                frame False {
                                n136 = call "readLightBarriersNew.vi"() -> ("light barriers"=w238:bool[])  [unwired: 1 out]
                                }
                                frame True {
                                n137 = global write "GlobalLB.vi" "LB status"("simulated LB status 5") -> ()
                                }
                                }
                                }
                                frame True {
                                n138 = global write "GlobalLB.vi" "LB status"("simulated LB status 2") -> ()
                                }
                                }
                                n139 = Index Array(array=w232, index=1) -> (element=w234:bool)
                                n140 = local write "light barriers"(w232) -> ()
                                n141 = node-c288() -> ()  [unwired: 1 in, 1 out]
                                }
                                n142 = node-c288(w230) -> ()  [unwired: 1 out]
                                }
                                }
                                }
                              }
                              n143 = local read "stop indicator"() -> (w180:bool)
                              n144 = Format Into String(format string="%d/%d", initial string="Sorting flies... " ("message"), w182, w185) -> (resulting string=w183:string)  [unwired: 1 in, 1 out]
                              n145 = Bundle By Name(cluster=cluster{"Program status":u32, "message":string} {"Program status"=0, "message"=""} ("status 2"), "Program status"=u32 6618880, "message"=w183) -> (w188:cluster{"Program status":u32, "message":string})
                              n146 = Or(x=w180, y=w181) -> (x .or. y?=w179:bool)
                              n147 = local write "status"(w188) -> ()
                            }
                          }
                          n148 = local write "measured flies"(w128) -> ()
                        }
                      }
                      frame #1 {
                        n149 = stacked-sequence {
                          tunnel: w248 -> [_ w253]
                          tunnel: w247 -> [_ w254]
                          frame #0 {
                            w249 = T4."Radio Selection 1" ("Robot Position")
                            n150 = local write "Robot Position"(w249) -> ()
                            n151 = call "RobotPosGUI.vi"("Robot Position"=w249) -> ("X position"=w251:i32, "Y position"=w250:i32)  [unwired: 4 in]
                            n152 = call "setPositionXY.vi"("Y Position"=w250, "X Position"=w251) -> ()  [unwired: 1 in]
                          }
                          frame #1 {
                            n153 = Increment(x=w253) -> (x+1=w252:i32)
                            n154 = local write "done sorting"(TRUE) -> ()
                            n155 = Format Into String(format string="%d/%d", initial string="Sorting flies... " ("message"), w252, w254) -> (resulting string=w260:string)  [unwired: 1 in, 1 out]
                            n156 = Bundle By Name(cluster=cluster{"Program status":u32, "message":string} {"Program status"=0, "message"=""} ("status 2"), "Program status"=u32 6618880, "message"=w260) -> (w256:cluster{"Program status":u32, "message":string})
                            n157 = local write "status"(w256) -> ()
                          }
                        }
                      }
                    }
                  }
                }
              }
            }
          }
          frame True {
            n158 = Tick Count (ms)() -> (millisecond timer value=w265:u32)
            "last time collected fly" <- w265
            n159 = node-c288(w269, 200 ("Priority"), nitl_modes."Process missed periods, ignore original phase" ("Mode")) -> (w275:T12)  [unwired: 1 in]
            n160 = timed-loop {
              shift-right: [w340] -> _
              shift-left: T3."blowing back" ("task control") -> [w338]
              shift-right: [w342] -> _
              shift-left: _ -> [w343]
              timing: w275 -> [_]
              timing-out: [_] -> w274
              shift-right: [w341] -> _
              shift-left: w265 -> [w344]
              i -> [w339]
              stop <- w345 stop-if-true
              n161 = node-c288() -> ()  [unwired: 1 in, 1 out]
              n162 = case shown="\"blowing back\"" w338 {
                tunnel: w344 -> [w348 _ _ w441 _ _ _]
                tunnel: [w350 T3."fly in chamber" w383 w439 T3."waiting for fly" T3."waiting for fly" T3."waiting for fly"] -> w340
                tunnel: [w349 w375 w397 w438 w480 w545 w595] -> w342
                tunnel: [w348 w375 w398 w441 w479 w546 w596] -> w341
                tunnel: w343 -> [w349 _ w397 w438 w480 w545 w595]
                frame "waiting for fly", Default {
                  n163 = case shown="False" "simulate LB" {
                    tunnel: [w353 "simulated LB status"] -> w346
                    frame False {
                      n164 = call "readLightBarriersNew.vi"() -> ("light barriers"=w353:bool[])  [unwired: 1 out]
                    }
                    frame True {
                      n165 = global write "GlobalLB.vi" "LB status"("simulated LB status") -> ()
                    }
                  }
                  "light barriers" <- w346
                  n166 = Index Array(array=w346, index=0) -> (element=w351:bool)
                  n167 = case shown="False" w351 {
                    tunnel: [w363 T3."closing gate"] -> w350
                    tunnel: w348 -> [w364 _]
                    frame False {
                      n168 = local read "last time collected fly"() -> (w357:u32)
                      n169 = Multiply(x="activate flies time interval (s)", y=u32 1000) -> (x*y=w367:u32)
                      n170 = Tick Count (ms)() -> (millisecond timer value=w355:u32)
                      n171 = Multiply(x="inactivity alarm time interval (s)", y=u32 1000) -> (x*y=w360:u32)
                      n172 = Subtract(x=w355, y=w357) -> (x-y=w358:u32)
                      n173 = Subtract(x=w355, y=w364) -> (x-y=w366:u32)
                      n174 = Less?(x=w366, y=w367) -> (x < y?=w365:bool)
                      n175 = Less?(x=w358, y=w360) -> (x < y?=w356:bool)
                      n176 = case shown="False" w356 {
                        tunnel: w355 -> [w369 _]
                        frame False {
                          n177 = local read "sounds"() -> (w370:T11)
                          n178 = call "playInactivitySound.vi"("sounds"=w370) -> ()  [unwired: 11 in]
                          n179 = local write "last time collected fly"(w369) -> ()
                        }
                        frame True {
                        }
                      }
                      n180 = case shown="True" w365 {
                        tunnel: [T3."activate flies" T3."waiting for fly"] -> w363
                        frame False {
                        }
                        frame True {
                        }
                      }
                    }
                    frame True {
                    }
                  }
                }
                frame "closing gate" {
                  n181 = flat-sequence {
                    frame #0 {
                      n182 = Wait (ms)(milliseconds to wait="milliseconds to wait\nafter detection") -> ()  [unwired: 1 out]
                    }
                    frame #1 {
                      n183 = local read "gate 0 closed"() -> (w377:u16)
                      n184 = call "setServoArduinoNew.vi"("speed"=u8 0, "Pulse Width in uS"=w377, "servo id"=u8 0 ("channel")) -> ()
                    }
                    frame #2 {
                      n185 = local read "fly sieve hangar"() -> (w382:u16)
                      n186 = call "setServoArduinoNew.vi"("speed"=u8 0, "Pulse Width in uS"=w382, "servo id"=u8 1 ("channel")) -> ()
                    }
                  }
                  n187 = Tick Count (ms)() -> (millisecond timer value=w375:u32)
                }
                frame "fly in chamber" {
                  n188 = global read "GlobalBaslerCamera.vi" "number of valid images acquired"() -> (w393:i32)
                  n189 = Multiply(x="max time \nin chamber after\ndetection (s)", y=u32 1000) -> (x*y=w389:u32)
                  n190 = Tick Count (ms)() -> (millisecond timer value=w398:u32)
                  n191 = Multiply(x="max time\nin chamber (s)", y=u32 1000) -> (x*y=w401:u32)
                  n192 = Greater Than 0?(x=w393) -> (x > 0?=w392:bool)
                  n193 = Subtract(x=w398, y=w397) -> (x-y=w385:u32)
                  n194 = Less?(x=w385, y=w389) -> (x < y?=w388:bool)
                  n195 = Less?(x=w385, y=w401) -> (x < y?=w394:bool)
                  n196 = And(x=w388, y=w392) -> (x .and. y?=w387:bool)
                  n197 = Or(x=w394, y=w387) -> (x .or. y?=w386:bool)
                  n198 = case shown="True" w386 {
                    tunnel: [T3."blowing back" w432] -> w384
                    tunnel: w393 -> [_ w427]
                    frame False {
                    }
                    frame True {
                      n199 = global read "GlobalBaslerCamera.vi" "touching rigth border"() -> (w428:bool)
                      n200 = Greater Or Equal?(x=w427, y="max number of\nimages per fly") -> (x >= y?=w429:bool)
                      n201 = Or(x=w428, y=w429) -> (x .or. y?=w430:bool)
                      n202 = case shown="False" w430 {
                        tunnel: [T3."fly in chamber" T3."taking decision"] -> w432
                        frame False {
                        }
                        frame True {
                        }
                      }
                    }
                  }
                  n203 = Equal?(x=w384, y=T3."fly in chamber") -> (x = y?=w395:bool)
                  n204 = case shown="True" w395 {
                    tunnel: w385 -> [_ w411]
                    tunnel: w384 -> [w402 w404]
                    tunnel: [w402 w403] -> w383
                    frame False {
                    }
                    frame True {
                      n205 = local read "simulate LB"() -> (w406:bool)
                      n206 = case shown="False" w406 {
                        tunnel: [w413 "simulated LB status 3"] -> w405
                        frame False {
                          n207 = call "readLightBarriersNew.vi"() -> ("light barriers"=w413:bool[])  [unwired: 1 out]
                        }
                        frame True {
                          n208 = global write "GlobalLB.vi" "LB status"("simulated LB status 3") -> ()
                        }
                      }
                      n209 = Index Array(array=w405, index=0) -> (element=w409:bool)
                      n210 = local write "light barriers"(w405) -> ()
                      n211 = Greater?(x=w411, y="insensitivity time (ms)") -> (0:w408:bool)
                      n212 = And(x=w408, y=w409) -> (x .and. y?=w407:bool)
                      n213 = case shown="True" w407 {
                        tunnel: w404 -> [w415 w417]
                        tunnel: [w415 w416] -> w403
                        frame False {
                        }
                        frame True {
                          n214 = Greater Than 0?(x="shakeSpan") -> (x > 0?=w419:bool)
                          n215 = case shown="False" w419 {
                            tunnel: "shakeSpan" -> [_ w422]
                            tunnel: w417 -> [_ w421]
                            tunnel: [T3."blowing back" w421] -> w416
                            frame False {
                            }
                            frame True {
                              n216 = call "shakeServoArduinoNew.vi"("milliseconds to wait"="shake speed", "numShakes"="numShakes", "shake span"=w422, "servo id"=u8 0 ("channel")) -> ()  [unwired: 8 in]
                            }
                          }
                        }
                      }
                    }
                  }
                }
                frame "taking decision" {
                  n217 = flat-sequence {
                    tunnel: w438 -> [w442]
                    tunnel: [w461] -> w437
                    tunnel: w437 -> [w463]
                    tunnel: [w463] -> w436
                    tunnel: w436 -> [w466]
                    tunnel: [w466] -> w435
                    tunnel: [w470] -> w440
                    tunnel: w435 -> [w467]
                    tunnel: [w478] -> w439
                    tunnel: w440 -> [w478]
                    frame #0 {
                      n218 = node-c288(i64 10 ("Period")) -> (w445:T12)  [unwired: 3 in]
                      n219 = timed-loop {
                        timing: w445 -> [_]
                        timing-out: [_] -> w444
                        tunnel: w442 -> [w446]
                        stop <- w449 stop-if-true
                        n220 = node-c288() -> ()  [unwired: 1 in, 1 out]
                        n221 = Tick Count (ms)() -> (millisecond timer value=w448:u32)
                        n222 = global read "GlobalBaslerCamera.vi" "filled buffer"() -> (w453:i32)
                        n223 = Subtract(x=w448, y=w446) -> (x-y=w447:u32)
                        n224 = Greater?(x=w447, y=u32 100) -> (0:w451:bool)
                        n225 = Equal To 0?(x=w453) -> (x = 0?=w452:bool)
                        n226 = And(x=w452, y=w451) -> (x .and. y?=w449:bool)
                        n227 = node-c288() -> ()  [unwired: 1 in, 1 out]
                      }
                      n228 = node-c288(w444) -> ()  [unwired: 1 out]
                    }
                    frame #1 {
                      n229 = call "extractBodyOpenCVIP.vi"("minImageNumber"="minimum valid\nimages per fly") -> ("found fly"=w461:bool)  [unwired: 2 in]
                    }
                    frame #2 {
                      n230 = Wait (ms)(milliseconds to wait=u32 350) -> ()  [unwired: 1 out]
                    }
                    frame #3 {
                      n231 = global read "GlobalBaslerCamera.vi" "temp path"() -> (w465:path)
                      n232 = call "getWSIOpenCVIP.vi"("File Path"=w465) -> ("Image Dst Out"=→"pre-processing result":T2)  [unwired: 1 in, 1 out]
                    }
                    frame #4 {
                      n233 = case shown="True" "keep all flies" {
                        tunnel: [w471 TRUE ("found fly")] -> w469
                        tunnel: w467 -> [w471 _]
                        frame False {
                        }
                        frame True {
                        }
                      }
                      n234 = case shown="True" w469 {
                        tunnel: [T3."blowing back" T3."keeping the fly"] -> w470
                        tunnel: "keep all flies" -> [_ _]
                        tunnel: w467 -> [_ w474]
                        frame False {
                        }
                        frame True {
                          n235 = case shown="True" w474 {
                            frame False {
                            }
                            frame True {
                              n236 = global read "GlobalBaslerCamera.vi" "temp path"() -> (w476:path)
                              n237 = call "writeBrightestToFile.vi"("base path"=w476) -> ()  [unwired: 11 in]
                            }
                          }
                        }
                      }
                    }
                    frame #5 {
                      n238 = global write "GlobalBaslerCamera.vi" "touching rigth border"(FALSE ("touching rigth border")) -> ()
                    }
                  }
                }
                frame "keeping the fly" {
                  n239 = flat-sequence {
                    frame #0 {
                      n240 = local read "numPuffs keep"() -> (w484:i32)
                      n241 = local read "valve open time keep"() -> (w483:u32)
                      n242 = local read "valves puffed"() -> (w487:bool[])
                      n243 = local read "valve close"() -> (w485:bool[])
                      n244 = call "setValvesPuffedArduinoNew.vi"("valve data puffed"=w487, "valve data close"=w485, "valve data open"="valve to hangar", "milliseconds to wait"=w483, "numPuffs"=w484) -> ()  [unwired: 7 in]
                    }
                    frame #1 {
                      n245 = Wait (ms)(milliseconds to wait=u32 150) -> ()  [unwired: 1 out]
                    }
                    frame #2 {
                      n246 = node-c288(i64 20 ("Period")) -> (w491:T12)  [unwired: 3 in]
                      n247 = timed-loop {
                        timing: w491 -> [_]
                        timing-out: [_] -> w490
                        stop <- w494 stop-if-true
                        n248 = node-c288() -> ()  [unwired: 1 in, 1 out]
                        n249 = local read "simulate LB"() -> (w493:bool)
                        n250 = case shown="False" w493 {
                          tunnel: [w496 "simulated LB status 4"] -> w492
                          frame False {
                            n251 = call "readLightBarriersNew.vi"() -> ("light barriers"=w496:bool[])  [unwired: 1 out]
                          }
                          frame True {
                            n252 = global write "GlobalLB.vi" "LB status"("simulated LB status 4") -> ()
                          }
                        }
                        n253 = local write "light barriers"(w492) -> ()
                        n254 = Index Array(array=w492, index=1) -> (element=w494:bool)
                        n255 = node-c288() -> ()  [unwired: 1 in, 1 out]
                      }
                      n256 = node-c288(w490) -> ()  [unwired: 1 out]
                    }
                    frame #3 {
                      n257 = global read "GlobalBaslerCamera.vi" "temp path"() -> (w505:path)
                      n258 = global read "GlobalBaslerCamera.vi" "data path"() -> (w504:path)
                      n259 = local read "Robot Position"() -> (w506:T4)
                      n260 = call "saveImageData.vi"("Robot Position 2"=w506, "data path"=w504, "temp path"=w505) -> ()  [unwired: 8 in, 1 out]
                    }
                    frame #4 {
                      n261 = call "setXYToNextPosition.vi"() -> ("X position"=w510:i32, "Y position"=w511:i32, "Robot Position"=w508:T4)  [unwired: 1 in]
                      n262 = Equal?(x=w508, y=T4."Radio Selection 1") -> (x = y?=w509:bool)
                      n263 = local write "Robot Position"(w508) -> ()
                      n264 = local write "measured flies"(w508) -> ()
                      n265 = case shown="True" w509 {
                        frame False {
                        }
                        frame True {
                          n266 = global write "GlobalStatus.vi" "hangar full"(TRUE ("hangar full")) -> ()
                        }
                      }
                      n267 = call "setPositionXY.vi"("Y Position"=w511, "X Position"=w510) -> ()  [unwired: 1 in]
                    }
                    frame #5 {
                      n268 = flat-sequence {
                        tunnel: [w516] -> w514
                        tunnel: w514 -> [w518]
                        tunnel: [w518] -> w513
                        tunnel: w513 -> [w522]
                        tunnel: [w522] -> w515
                        tunnel: w515 -> [w523]
                        frame #0 {
                          n269 = global read "OpenCvGlobals.vi" "opencv semaphore"() -> (w517:T16)
                          n270 = call <vilib>:"Acquire Semaphore.vi"("semaphore"=w517) -> ("semaphore out"=w516:T16)  [unwired: 4 in, 2 out]
                        }
                        frame #1 {
                          n271 = call "cleanUpOpenCVIP.vi"() -> ()  [unwired: 4 in, 1 out]
                        }
                        frame #2 {
                          n272 = global read "GlobalBaslerCamera.vi" "temp path"() -> (w520:path)
                          n273 = local read "Image processing preferences"() -> (w521:T1)
                          n274 = Path To String(path=w520) -> (string=w519:string)
                          n275 = call "InitializeOpenCVIP.vi"("dataDirectory"=w519, "Image processing preferences"=w521) -> ()  [unwired: 1 out]
                        }
                        frame #3 {
                          n276 = call <vilib>:"Release Semaphore.vi"("semaphore"=w523) -> ()  [unwired: 5 in, 2 out]
                        }
                      }
                    }
                    frame #6 {
                      n277 = local read "fly sieve odour"() -> (w524:u16)
                      n278 = call "setServoArduinoNew.vi"("speed"=u8 0, "Pulse Width in uS"=w524, "servo id"=u8 1 ("channel")) -> ()
                      n279 = case shown="True" "free gate after keeping" {
                        frame False {
                          n280 = local read "gate 0 open"() -> (w530:u16)
                          n281 = call "setServoArduinoNew.vi"("speed"=u8 0, "Pulse Width in uS"=w530, "servo id"=u8 0 ("channel")) -> ()
                        }
                        frame True {
                          n282 = stacked-sequence {
                            frame #0 {
                              n283 = local read "gate 0 open blowing"() -> (w531:u16)
                              n284 = call "setServoArduinoNew.vi"("speed"=u8 0, "Pulse Width in uS"=w531, "servo id"=u8 0 ("channel")) -> ()
                            }
                            frame #1 {
                              n285 = local read "valves puffed"() -> (w538:bool[])
                              n286 = local read "valve close"() -> (w537:bool[])
                              n287 = local read "valve back"() -> (w534:bool[])
                              n288 = call "setValvesPuffedArduinoNew.vi"("valve data puffed"=w538, "valve data close"=w537, "valve data open"=w534, "milliseconds to wait"=u32 200, "numPuffs"=1) -> ()  [unwired: 7 in]
                            }
                            frame #2 {
                              n289 = local read "gate 0 open"() -> (w539:u16)
                              n290 = call "setServoArduinoNew.vi"("speed"=u8 30, "Pulse Width in uS"=w539, "servo id"=u8 0 ("channel")) -> ()
                            }
                          }
                        }
                      }
                    }
                    frame #7 {
                      # "force background save"
                      n291 = global write "GlobalBaslerCamera.vi" "force background save"(TRUE ("force background save")) -> ()
                      n292 = Wait (ms)(milliseconds to wait=u32 150) -> ()  [unwired: 1 out]
                    }
                  }
                  n293 = global write "GlobalBaslerCamera.vi" "number of valid images acquired"(0 ("number of valid images acquired")) -> ()
                  n294 = Tick Count (ms)() -> (millisecond timer value=w479:u32)
                  n295 = local write "last time collected fly"(w479) -> ()
                }
                frame "blowing back" {
                  n296 = flat-sequence {
                    frame #0 {
                      n297 = local read "fly sieve back"() -> (w548:u16)
                      n298 = call "setServoArduinoNew.vi"("speed"=u8 0, "Pulse Width in uS"=w548, "servo id"=u8 1 ("channel")) -> ()
                    }
                    frame #1 {
                      # "was waiting\n2500ms"
                      n299 = Wait (ms)(milliseconds to wait=u32 300) -> ()  [unwired: 1 out]
                    }
                    frame #2 {
                      n300 = local read "gate 0 open blowing"() -> (w552:u16)
                      n301 = local read "fly trap open"() -> (w553:u16)
                      n302 = call "setServoArduinoNew.vi"("speed"=u8 0, "Pulse Width in uS"=w552, "servo id"=u8 0 ("channel")) -> ()
                      n303 = call "setServoArduinoNew.vi"("speed"=u8 0, "Pulse Width in uS"=w553, "servo id"=u8 3 ("channel")) -> ()
                    }
                    frame #3 {
                      n304 = local read "valve back"() -> (w562:bool[])
                      n305 = local read "numPuffs blowback"() -> (w558:i32)
                      n306 = call "resetTempFolder.vi"() -> ()  [unwired: 12 in]
                      n307 = local read "valve close"() -> (w560:bool[])
                      n308 = local read "valve close"() -> (w561:bool[])
                      n309 = call "setValvesPuffedArduinoNew.vi"("valve data puffed"=w561, "valve data close"=w560, "valve data open"=w562, "milliseconds to wait"="valve open time blow back", "numPuffs"=w558) -> ()  [unwired: 7 in]
                    }
                    frame #4 {
                      n310 = call "setServoArduinoNew.vi"("speed"=u8 0, "Pulse Width in uS"="gate 0 closed blowing", "servo id"=u8 0 ("channel")) -> ()
                    }
                    frame #5 {
                      n311 = Wait (ms)(milliseconds to wait=u32 200) -> ()  [unwired: 1 out]
                    }
                    frame #6 {
                      n312 = local read "valve back"() -> (w568:bool[])
                      n313 = local read "valve close"() -> (w570:bool[])
                      n314 = local read "valves puffed"() -> (w569:bool[])
                      n315 = call "setValvesPuffedArduinoNew.vi"("valve data puffed"=w569, "valve data close"=w570, "valve data open"=w568, "milliseconds to wait"="valve open time blow back 2", "numPuffs"=1) -> ()  [unwired: 7 in]
                    }
                    frame #7 {
                      n316 = local read "fly sieve odour"() -> (w578:u16)
                      n317 = local read "fly trap close"() -> (w572:u16)
                      n318 = local read "gate 0 open"() -> (w575:u16)
                      n319 = call "setServoArduinoNew.vi"("speed"=u8 0, "Pulse Width in uS"=w578, "servo id"=u8 1 ("channel")) -> ()
                      n320 = call "setServoArduinoNew.vi"("speed"=u8 30, "Pulse Width in uS"=w572, "servo id"=u8 3 ("channel")) -> ()
                      n321 = call "setServoArduinoNew.vi"("speed"=u8 30, "Pulse Width in uS"=w575, "servo id"=u8 0 ("channel")) -> ()
                    }
                    frame #8 {
                      n322 = flat-sequence {
                        tunnel: [w584] -> w582
                        tunnel: w582 -> [w586]
                        tunnel: [w586] -> w581
                        tunnel: w581 -> [w590]
                        tunnel: [w590] -> w583
                        tunnel: w583 -> [w591]
                        frame #0 {
                          n323 = global read "OpenCvGlobals.vi" "opencv semaphore"() -> (w585:T16)
                          n324 = call <vilib>:"Acquire Semaphore.vi"("semaphore"=w585) -> ("semaphore out"=w584:T16)  [unwired: 4 in, 2 out]
                        }
                        frame #1 {
                          n325 = call "cleanUpOpenCVIP.vi"() -> ()  [unwired: 4 in, 1 out]
                        }
                        frame #2 {
                          n326 = global read "GlobalBaslerCamera.vi" "temp path"() -> (w588:path)
                          n327 = local read "Image processing preferences"() -> (w589:T1)
                          n328 = Path To String(path=w588) -> (string=w587:string)
                          n329 = call "InitializeOpenCVIP.vi"("dataDirectory"=w587, "Image processing preferences"=w589) -> ()  [unwired: 1 out]
                        }
                        frame #3 {
                          n330 = call <vilib>:"Release Semaphore.vi"("semaphore"=w591) -> ()  [unwired: 5 in, 2 out]
                        }
                      }
                    }
                    frame #9 {
                      n331 = global write "GlobalBaslerCamera.vi" "force background save"(TRUE ("force background save")) -> ()
                      n332 = Wait (ms)(milliseconds to wait=u32 150) -> ()  [unwired: 1 out]
                    }
                  }
                  n333 = global write "GlobalBaslerCamera.vi" "number of valid images acquired"(0 ("number of valid images acquired")) -> ()
                  n334 = Tick Count (ms)() -> (millisecond timer value=w546:u32)
                }
                frame "activate flies" {
                  n335 = flat-sequence {
                    tunnel: [w635] -> w596
                    frame #0 {
                      n336 = local read "fly sieve back"() -> (w600:u16)
                      n337 = local read "fly trap open"() -> (w597:u16)
                      n338 = call "setServoArduinoNew.vi"("speed"=u8 0, "Pulse Width in uS"=w597, "servo id"=u8 3 ("channel")) -> ()
                      n339 = call "setServoArduinoNew.vi"("speed"=u8 0, "Pulse Width in uS"=w600, "servo id"=u8 1 ("channel")) -> ()
                    }
                    frame #1 {
                      # "was waiting\n2500ms"
                      n340 = Wait (ms)(milliseconds to wait=u32 200) -> ()  [unwired: 1 out]
                    }
                    frame #2 {
                      n341 = stacked-sequence {
                        frame #0 {
                          n342 = local read "valve close"() -> (w605:bool[])
                          n343 = local read "valve back"() -> (w606:bool[])
                          n344 = call "setValvesArduinosSinglePuffNew.vi"("milliseconds to wait"="valve open time activate pre", "valve data close"=w605, "valve data open"=w606) -> ()  [unwired: 9 in]
                        }
                        frame #1 {
                          n345 = Wait (ms)(milliseconds to wait=u32 200) -> ()  [unwired: 1 out]
                        }
                        frame #2 {
                          n346 = local read "gate 0 closed blowing"() -> (w610:u16)
                          n347 = call "setServoArduinoNew.vi"("speed"=u8 0, "Pulse Width in uS"=w610, "servo id"=u8 0 ("channel")) -> ()
                        }
                        frame #3 {
                          n348 = Subtract(x="number of\npuffs for scaring", y=1) -> (x-y=w613:i32)
                          n349 = for {
                            N: w613 -> [_]
                            n350 = local read "valve close"() -> (w615:bool[])
                            n351 = local read "valve back"() -> (w616:bool[])
                            n352 = call "setValvesArduinosSinglePuffNew.vi"("milliseconds to wait"="valve open time activate", "valve data close"=w615, "valve data open"=w616) -> ()  [unwired: 9 in]
                          }
                        }
                      }
                    }
                    frame #3 {
                      n353 = stacked-sequence {
                        frame #0 {
                          n354 = local read "gate 0 open blowing"() -> (w620:u16)
                          n355 = local read "fly trap close"() -> (w617:u16)
                          n356 = call "setServoArduinoNew.vi"("speed"=u8 0, "Pulse Width in uS"=w620, "servo id"=u8 0 ("channel")) -> ()
                          n357 = call "setServoArduinoNew.vi"("speed"=u8 30, "Pulse Width in uS"=w617, "servo id"=u8 3 ("channel")) -> ()
                        }
                        frame #1 {
                          n358 = Wait (ms)(milliseconds to wait=u32 500) -> ()  [unwired: 1 out]
                        }
                        frame #2 {
                          n359 = local read "valves puffed"() -> (w628:bool[])
                          n360 = local read "valve close"() -> (w627:bool[])
                          n361 = local read "valve back"() -> (w624:bool[])
                          n362 = call "setValvesPuffedArduinoNew.vi"("valve data puffed"=w628, "valve data close"=w627, "valve data open"=w624, "milliseconds to wait"=u32 200, "numPuffs"=1) -> ()  [unwired: 7 in]
                        }
                        frame #3 {
                          n363 = local read "gate 0 open"() -> (w629:u16)
                          n364 = call "setServoArduinoNew.vi"("speed"=u8 0, "Pulse Width in uS"=w629, "servo id"=u8 0 ("channel")) -> ()
                        }
                      }
                    }
                    frame #4 {
                      n365 = local read "fly sieve odour"() -> (w636:u16)
                      n366 = local read "gate 0 open"() -> (w632:u16)
                      n367 = call "setServoArduinoNew.vi"("speed"=u8 0, "Pulse Width in uS"=w632, "servo id"=u8 0 ("channel")) -> ()
                      n368 = call "setServoArduinoNew.vi"("speed"=u8 0, "Pulse Width in uS"=w636, "servo id"=u8 1 ("channel")) -> ()
                      n369 = Tick Count (ms)() -> (millisecond timer value=w635:u32)
                    }
                  }
                }
              }
              n370 = local read "stop indicator"() -> (w345:bool)
              n371 = node-c288() -> ()  [unwired: 1 in, 1 out]
              "task out" <- w338
              "numCycles" <- w339
            }
            n372 = while {
              i -> [w276]
              stop <- w277 stop-if-true
              n373 = event shown="[0] Timeout" {
                selector: _ -> [_ _ _ _ _]
                dyn-events: _ -> [_ _ _ _ _]
                timeout: 20 -> [_ _ _ _ _]
                event Timeout {
                  n374 = event-data() -> ()  [unwired: 1 in, 2 out]
                }
                event "image selector": Value Change {
                  n375 = event-data() -> ("NewVal"=w280:u16)  [unwired: 1 in]
                  n376 = Less?(x=w280, y=u16 5) -> (x < y?=w281:bool)
                  n377 = case shown="True" w281 {
                    tunnel: [w283 w284] -> w282
                    frame False {
                      w283 = u32 1 items=["Grayscale", "Binary", "Gradient", "Rainbow", "Temperature", "User Defined"] ("Palette:Palette Type")
                    }
                    frame True {
                      w284 = u32 0 items=["Grayscale", "Binary", "Gradient", "Rainbow", "Temperature", "User Defined"] ("Palette:Palette Type")
                    }
                  }
                  n378 = property on="image" class="ImageControl"("Palette Type"=w282) -> ()  [unwired: 2 in, 2 out]
                }
                event "adjust image": Value Change {
                  n379 = event-data() -> ("NewVal"=w285:bool)  [unwired: 1 in]
                  n380 = case shown="True" w285 {
                    frame False {
                      n381 = local read "gate 0 open"() -> (w288:u16)
                      n382 = call "setServoArduinoNew.vi"("speed"=u8 0, "Pulse Width in uS"=w288, "servo id"=u8 0 ("channel")) -> ()
                    }
                    frame True {
                      n383 = local read "gate 0 closed"() -> (w291:u16)
                      n384 = call "setServoArduinoNew.vi"("speed"=u8 0, "Pulse Width in uS"=w291, "servo id"=u8 0 ("channel")) -> ()
                    }
                  }
                  n385 = global write "GlobalBaslerCamera.vi" "adjust image"(w285) -> ()
                }
                event "valve open time keep": Value Change {
                  n386 = event-data() -> ("NewVal"=w292:u32)  [unwired: 1 in, 4 out]
                  n387 = global write "GlobalValves.vi" "valve open time"(w292) -> ()
                }
                event "open valve": Value Change {
                  n388 = event-data() -> ()  [unwired: 1 in, 5 out]
                  n389 = global read "GlobalValves.vi" "valve open time"() -> (w293:u32)
                  n390 = call "setValvesArduinosSinglePuffNew.vi"("milliseconds to wait"=w293, "valve data close"=bool[] [FALSE, FALSE, FALSE, FALSE, FALSE, FALSE, FALSE, FALSE] ("valve close 3"), "valve data open"=bool[] [TRUE, TRUE, FALSE, FALSE, FALSE, FALSE, FALSE, FALSE] ("valve open 3")) -> ()  [unwired: 9 in]
                }
              }
              n391 = local read "stop indicator"() -> (w277:bool)
              "events check loop" <- w276
            }
            n392 = node-c288(w274) -> ()  [unwired: 1 out]
            n393 = node-c288(i64 20 ("Period")) -> (w273:T12)  [unwired: 3 in]
            n394 = timed-loop {
              timing: w273 -> [_]
              timing-out: [_] -> w272
              shift-right: [w317] -> _
              shift-left: _ -> [w318]
              stop <- w325 stop-if-true
              n395 = node-c288() -> ()  [unwired: 1 in, 1 out]
              n396 = local read "task out"() -> (w317:T3)
              n397 = property on="task out" class="Enum (strict)"() -> ("Strings []"=w321:string[])  [unwired: 2 in, 2 out]
              n398 = global read "GlobalBaslerCamera.vi" "filled buffer"() -> (→"filled buffer":i32)
              n399 = global read "GlobalValves.vi" "valves status"() -> (→"valves status":bool[])
              n400 = global read "GlobalBaslerCamera.vi" "saving background"() -> (→"saving background":bool)
              n401 = global read "GlobalBaslerCamera.vi" "touching rigth border"() -> (→"touching rigth border":bool)
              n402 = Not Equal?(x=w317, y=w318) -> (x != y?=w319:bool)
              n403 = case shown="True" w319 {
                tunnel: w317 -> [_ w330]
                frame False {
                }
                frame True {
                  n404 = call "playSounds.vi"("sounds"="sounds", "task"=w330) -> ()  [unwired: 1 in]
                }
              }
              n405 = Index Array(array=w321, index=w317) -> (element=w320:string)
              n406 = local read "status"() -> (w322:cluster{"Program status":u32, "message":string})
              n407 = Bundle By Name(cluster=w322, "Program status"=u32 6618880, "message"=w320) -> (w323:cluster{"Program status":u32, "message":string})
              n408 = local read "stop indicator"() -> (w325:bool)
              n409 = local write "status"(w323) -> ()
              n410 = node-c288() -> ()  [unwired: 1 in, 1 out]
            }
            n411 = node-c288(i64 20 ("Period")) -> (w271:T12)  [unwired: 3 in]
            n412 = timed-loop {
              timing: w271 -> [_]
              timing-out: [_] -> w270
              stop <- w299 stop-if-true
              n413 = node-c288() -> ()  [unwired: 1 in, 1 out]
              n414 = global read "GlobalBaslerCamera.vi" "image buffering semaphore"() -> (w298:T16)
              n415 = call <vilib>:"Get Semaphore Status.vi"("semaphore"=w298) -> ("# available"=w296:i32)  [unwired: 5 in, 5 out]
              n416 = Greater Than 0?(x=w296) -> (x > 0?=w297:bool)
              n417 = case shown="True" w297 {
                frame False {
                }
                frame True {
                  n418 = call "saveImages.vi"() -> ()  [unwired: 12 in]
                }
              }
              n419 = local read "stop indicator"() -> (w299:bool)
              n420 = node-c288() -> ()  [unwired: 1 in, 1 out]
            }
            n421 = node-c288(w272) -> ()  [unwired: 1 out]
            n422 = call "initImageCluster.vi"() -> ("output cluster"=w268:T18)  [unwired: 5 in]
            n423 = node-c288(w270) -> ()  [unwired: 1 out]
            n424 = while {
              tunnel: w268 -> [w315]
              stop <- w308 stop-if-true
              # "image processing loop"
              n425 = local read "image format controls"() -> (w306:T9)
              n426 = local read "task out"() -> (w307:T3)
              n427 = call "flyVideoAcquisition.vi"("image format controls"=w306, "image selector"="image selector", "resave BG time"="resave BG time", "image cluster"=w315, "im proc controls"="im proc controls", "status"=w307) -> ("image out"=→"image":T2, "processed FPS"=→"processed FPS":dbl, "acquired FPS"=→"acquired FPS":dbl, "acquiring video"=→"acquiring video":bool)  [unwired: 2 in]
              n428 = local read "stop indicator"() -> (w308:bool)
            }
          }
        }
      }
      frame #5 {
        n429 = local read "gate 0 closed"() -> (w657:u16)
        n430 = local read "fly sieve odour"() -> (w652:u16)
        n431 = local read "fly trap open"() -> (w649:u16)
        n432 = local read "manualStopIndicator"() -> (w647:bool)
        n433 = local read "sounds"() -> (w648:T11)
        n434 = call "setServoArduinoNew.vi"("speed"=u8 0, "Pulse Width in uS"=w652, "servo id"=u8 1 ("channel")) -> ()
        n435 = call "setServoArduinoNew.vi"("speed"=u8 0, "Pulse Width in uS"=w657, "servo id"=u8 0 ("channel")) -> ()
        n436 = call "setServoArduinoNew.vi"("speed"=u8 30, "Pulse Width in uS"=w649, "servo id"=u8 3 ("channel")) -> ()
        n437 = call "playFinishSound.vi"("manual stop"=w647, "sounds"=w648) -> ()  [unwired: 10 in]
      }
      frame #6 {
        w663 = T17."Enabled" ("Disabled")
        n438 = stacked-sequence {
          frame #0 {
            n439 = call "RobotPosGUI.vi"("Robot Position"=T4."Radio Selection 1") -> ("X position"=w668:i32, "Y position"=w667:i32)  [unwired: 4 in]
            n440 = call "setPositionXY.vi"("Y Position"=w667, "X Position"=w668) -> ()  [unwired: 1 in]
          }
          frame #1 {
            n441 = call "stopXYStage.vi"() -> ()  [unwired: 12 in]
          }
        }
        n442 = flat-sequence {
          frame #0 {
            n443 = local read "disable servo delay (ms)"() -> (w665:u32)
            n444 = Wait (ms)(milliseconds to wait=w665) -> ()  [unwired: 1 out]
          }
          frame #1 {
            n445 = call "disableServosArduinoNew.vi"() -> ()  [unwired: 1 in]
          }
          frame #2 {
            n446 = call "closeArduinoNew.vi"() -> ()  [unwired: 12 in]
          }
        }
        n447 = property on="stop" class="Bool (strict)"("Value"=FALSE ("stop")) -> ()  [unwired: 2 in, 2 out]
        n448 = local read "task"() -> (w660:bool)
        n449 = property on="loop period (ms)" class="DigNum (strict)"("DisabledEnum"=w663) -> ()  [unwired: 2 in, 2 out]
        n450 = property on="camera controls" class="Clust (strict)"("DisabledEnum"=w663) -> ()  [unwired: 2 in, 2 out]
        n451 = property on="image format controls" class="Clust (strict)"("DisabledEnum"=w663) -> ()  [unwired: 2 in, 2 out]
        n452 = property on="temp path" class="Path"("DisabledEnum"=w663) -> ()  [unwired: 2 in, 2 out]
        n453 = property on="data path" class="Path"("DisabledEnum"=w663) -> ()  [unwired: 2 in, 2 out]
        n454 = case shown="True" w660 {
          frame False {
          }
          frame True {
            n455 = call "stopBaslerCamera.vi"() -> ()  [unwired: 12 in]
            n456 = call "cleanUpOpenCVIP.vi"() -> ()  [unwired: 4 in, 1 out]
          }
        }
        n457 = property on="stop" class="Bool (strict)"("BoolText.Text"="START" ("Boolean Text.Text")) -> ()  [unwired: 2 in, 2 out]
        n458 = local read "status"() -> (w659:cluster{"Program status":u32, "message":string})
        n459 = Bundle By Name(cluster=w659, "Program status"=u32 0) -> (w661:cluster{"Program status":u32, "message":string})
        n460 = local write "status"(w661) -> ()
      }
    }
  }
